vi "Interrupt.vi"(8 "error in (no error)":errorcluster, 11 "Sequencer Core in":refnum<class "Sequencer Core.lvclass">) -> (0 "error out":errorcluster, 3 "Sequencer Core out":refnum<class "Sequencer Core.lvclass">)   [LabVIEW 2020, in "Sequencer.lvlib" / "Sequencer Core.lvclass"]
doc: "Send a notification on the Interrupt Notifier."
uses:
  Sequencer Core.lvclass
  Sequencer Core.lvclass/Sequencer Core.ctl
  PPL/HDH.Data.Generic.lvlibp/Synchronization/Notifier/Notifier.lvclass
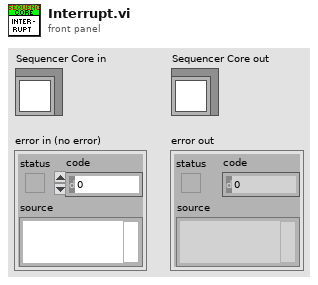
[diagram p1: front panel]
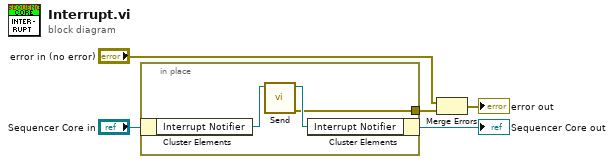
[diagram p0: block diagram]
diagram:
  n1 = in-place {
    in-place-border: [w6] -> w3
    n2 = in-place-cluster #1("Sequencer Core in") -> ("Interrupt Notifier"=w8:refnum<class "Notifier.lvclass">)
    n3 = call "Send.vi"("Notifier in"=w8) -> ("error out"=w6:errorcluster, "Notifier out"=w7:refnum<class "Notifier.lvclass">)  [unwired: 9 in]
    n4 = in-place-cluster #1("Interrupt Notifier"=w7) -> (→"Sequencer Core out":refnum<class "Sequencer Core.lvclass">)
  }
  n5 = Merge Errors("error in (no error)", w3) -> (→"error out":errorcluster)
